vi "HAL.vi"   [LabVIEW 2016]
uses:
  PLC/PLC.lvlib
types:
  T1 = cluster{"水样测试量程模式":enum16{"H", "L", "AUTO"}, "空白核查量程模式":enum16{"H", "L", "AUTO"}, "跨度核查量程模式":enum16{"H", "L", "AUTO"}, "加标回收量程模式":enum16{"H", "L", "AUTO"}}
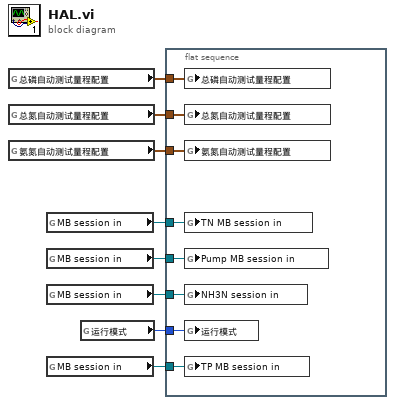
[diagram p0: block diagram]
diagram:
  n1 = global read "总磷总氮断电保存全局变量.vi" "总磷自动测试量程配置"() -> (w2:T1)
  n2 = global read "总磷总氮断电保存全局变量.vi" "总氮自动测试量程配置"() -> (w3:T1)
  n3 = global read "总磷总氮断电保存全局变量.vi" "氨氮自动测试量程配置"() -> (w1:T1)
  n4 = global read "VAR总磷总氮全局变量.vi" "MB session in"() -> (w4:refnum<class "MB_Master.lvclass">)
  n5 = global read "采配水全局变量.vi" "MB session in"() -> (w6:refnum<class "MB_Master.lvclass">)
  n6 = global read "VAR总磷总氮全局变量.vi" "MB session in"() -> (w7:refnum<class "MB_Master.lvclass">)
  n7 = global read "VAR总磷总氮全局变量.vi" "MB session in"() -> (w5:refnum<class "MB_Master.lvclass">)
  n8 = global read "系统设置全局变量.vi" "运行模式"() -> (w8:enum16{"维护模式", "常规模式", "应急模式", "质控模式"})
  n9 = flat-sequence {
    tunnel: w8 -> [w16]
    tunnel: w7 -> [w15]
    tunnel: w6 -> [w14]
    tunnel: w5 -> [w13]
    tunnel: w4 -> [w12]
    tunnel: w3 -> [w11]
    tunnel: w2 -> [w10]
    tunnel: w1 -> [w9]
    frame #0 {
      n10 = global write "系统交互.vi" "总磷自动测试量程配置"(w10) -> ()
      n11 = global write "系统交互.vi" "总氮自动测试量程配置"(w11) -> ()
      n12 = global write "系统交互.vi" "氨氮自动测试量程配置"(w9) -> ()
      n13 = global write "系统交互.vi" "TN MB session in"(w12) -> ()
      n14 = global write "系统交互.vi" "Pump MB session in"(w14) -> ()
      n15 = global write "系统交互.vi" "NH3N session in"(w15) -> ()
      n16 = global write "系统交互.vi" "运行模式"(w16) -> ()
      n17 = global write "系统交互.vi" "TP MB session in"(w13) -> ()
    }
  }
